vi "Set SysDef Path.vi"(10 "SysDef Path":path, 11 "Scalar Channels Testing in":refnum<class "FPGA Addon Test Class.lvclass">) -> (3 "Scalar Channels Testing out":refnum<class "FPGA Addon Test Class.lvclass">)   [LabVIEW 2018, in "FPGA Addon Test Class.lvclass"]
uses:
  FPGA Addon Test Class.lvclass
  FPGA Addon Test Class.lvclass/FPGA Addon Test Class.ctl
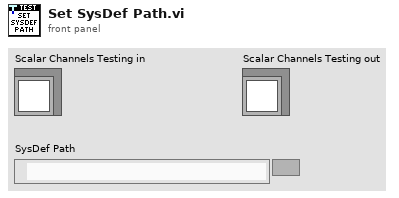
[diagram p1: front panel]
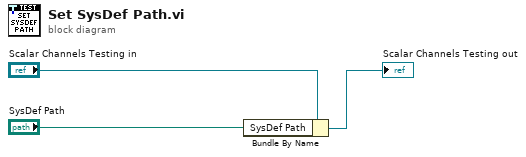
[diagram p0: block diagram]
diagram:
  n1 = Bundle By Name(cluster="Scalar Channels Testing in", "SysDef Path"="SysDef Path") -> (→"Scalar Channels Testing out":refnum<class "FPGA Addon Test Class.lvclass">)
